vi "Setup.vi"(8 "error in (no error)":errorcluster) -> (0 "error out":errorcluster, 3 "Bus Monitor out":refnum<class "Bus Monitor.lvclass">)   [LabVIEW 2020, in "Unit Tests.lvlib" / "Bus Monitor.lvclass"]
uses:
  Bus Monitor.lvclass
  Bus Monitor.lvclass/Bus Monitor.ctl
  Utilities/Simulated FPGA/FPGA Sim.lvclass
  C:/Users/MattJ/Desktop/git/bci-1553-labview-api/src/Dependencies/FPGA Interface/FPGA Interface.lvclass
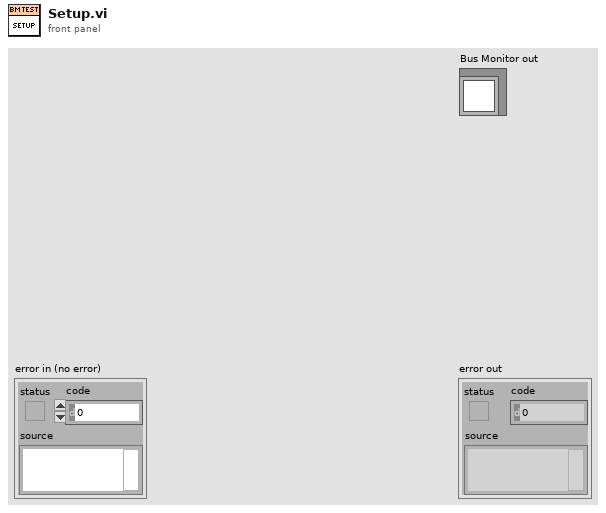
[diagram p1: front panel]
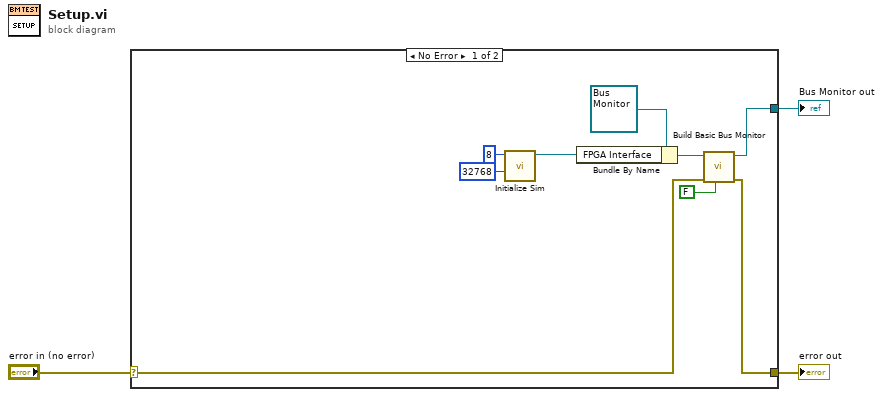
[diagram p0: block diagram]
diagram:
  n1 = case shown="No Error" "error in (no error)" {
    selector: "error in (no error)" -> [w6 w13]
    tunnel: [w5 w13] -> w2
    tunnel: [w7 _] -> w1
    frame No Error {
      n2 = call "Initialize Sim.vi"("Memory Size (32k)"=32768, "Components (8)"=8) -> ("FPGA Sim out"=w11:refnum<class "FPGA Sim.lvclass">)  [unwired: 8 in, 1 out]
      n3 = Bundle By Name(cluster=refnum<class "Bus Monitor.lvclass"> refnum ("Bus Monitor in"), "FPGA Interface"=w11) -> (w8:refnum<class "Bus Monitor.lvclass">)
      n4 = call "Build Basic Bus Monitor.vi"("48-bit Time Tag"=FALSE, "error in (no error)"=w6, "Bus Monitor in"=w8) -> ("error out"=w5:errorcluster, "Bus Monitor out"=w7:refnum<class "Bus Monitor.lvclass">)  [unwired: 7 in]
    }
    frame Error {
    }
  }
  "error out" <- w2
  "Bus Monitor out" <- w1
